vi "Write Ports Array.vi"(8 "error in (no error)":errorcluster, 10 "Array INP":cluster{"String":string, "Array 2":bool[]}[](array[cluster]), 11 "Ports in":refnum<class "Ports.lvclass">) -> (0 "error out":errorcluster, 3 "Ports out":refnum<class "Ports.lvclass">)   [LabVIEW 2010, in "Ports.lvclass"]
uses:
  Ports.lvclass
  Ports.lvclass/Ports.ctl
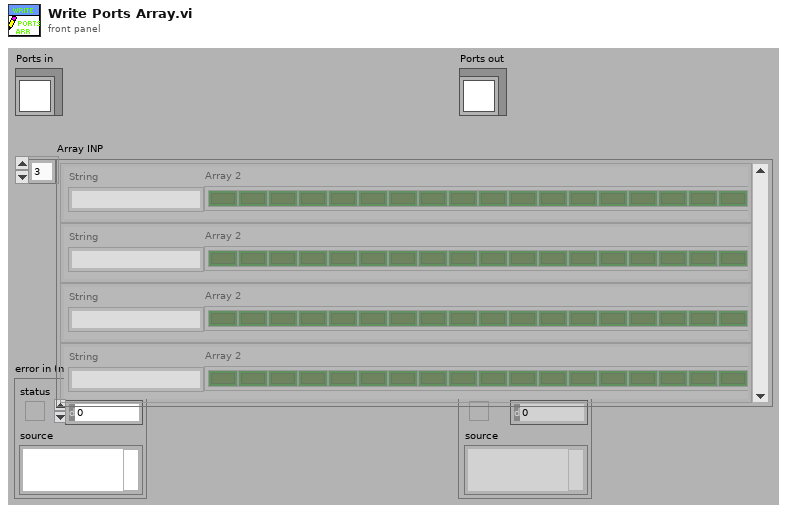
[diagram p1: front panel]
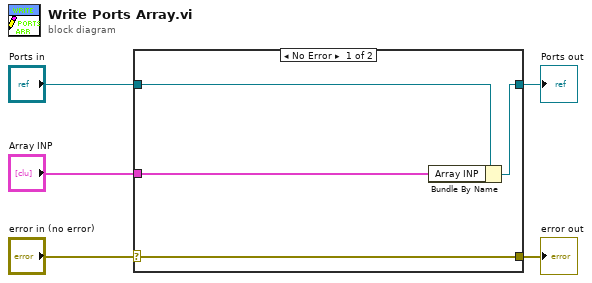
[diagram p0: block diagram]
diagram:
  n1 = case shown="No Error" "error in (no error)" {
    selector: "error in (no error)" -> [w9 w10]
    tunnel: [w9 w10] -> w4
    tunnel: [w7 w11] -> w2
    tunnel: "Ports in" -> [w8 w11]
    tunnel: "Array INP" -> [w6 _]
    frame No Error {
      n2 = Bundle By Name(cluster=w8, "Array INP"=w6) -> (w7:refnum<class "Ports.lvclass">)
    }
    frame Error {
    }
  }
  "error out" <- w4
  "Ports out" <- w2
